vi "Get Name.vi"(8 "error in (no error)":errorcluster, 11 "Dependency Source_Custom in":refnum<class "Dependency Source_Custom.lvclass">) -> (0 "error out":errorcluster, 2 "Dependency Source Name":string, 3 "Dependency Source_Custom out":refnum<class "Dependency Source_Custom.lvclass">)   [LabVIEW 2019, in "Project.Dependencies Finder.lvlib" / "Dependency Source_Custom.lvclass"]
doc: "Return the name of the dependency source. \n\nOnly non-empty strings are valid."
uses:
  Dependency Source_Custom.lvclass
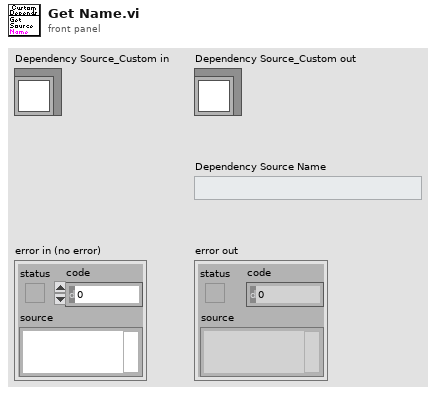
[diagram p1: front panel]
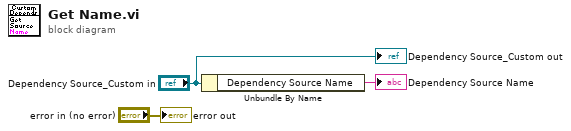
[diagram p0: block diagram]
diagram:
  n1 = Unbundle By Name("Dependency Source_Custom in") -> ("Dependency Source Name"=→"Dependency Source Name":string)
  "error out" <- "error in (no error)"
  "Dependency Source_Custom out" <- "Dependency Source_Custom in"
